vi "FGV_EXIT.vi"(4 "Function":enum16{"Read", "Write"}(ring), 6 "EXIT":bool caption="Abort") -> (1 "EXIT out":bool)   [LabVIEW 2019]
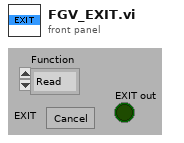
[diagram p1: front panel]
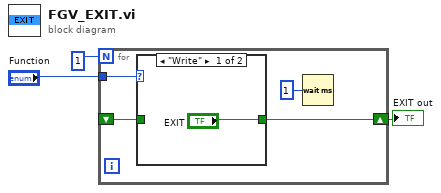
[diagram p0: block diagram]
diagram:
  n1 = for {
    N: 1 -> [_]
    shift-right: [w6] -> w2
    shift-left: _ -> [w7]
    tunnel: "Function" -> [w5]
    n2 = case shown="\"Write\"" w5 {
      tunnel: w7 -> [_ w9]
      tunnel: ["EXIT" w9] -> w6
      frame "Write" {
      }
      frame "Read", Default {
      }
    }
    n3 = Wait (ms)(milliseconds to wait=u32 1) -> ()  [unwired: 1 out]
  }
  "EXIT out" <- w2
